vi "Cmd_U32U32U32U32U32U32U32U32U8.vi"(0 "VISA Refnum in":refnum<visa-resource-name>, 1 "Arg1":u32 max=127 step=1, 2 "Arg2":u32 max=127 step=1, 3 "Arg3":u32, 5 "Address":u8, 7 "Cmd":u8, 8 "Arg4":u32, 9 "Arg9":u8, 10 "Arg5":u32, 11 "error in (no error)":errorcluster, 12 "Arg8":u32, 13 "Arg7":u32, 14 "Arg6":u32) -> (4 "VISA Refnum out":refnum<visa-resource-name>, 6 "Valid":bool, 15 "error out":errorcluster)   [LabVIEW 2015, in "Ion Motion Roboclaw.lvlib"]
uses:
  <instrlib>/Ion Motion Roboclaw/Ion Motion Roboclaw.lvlib
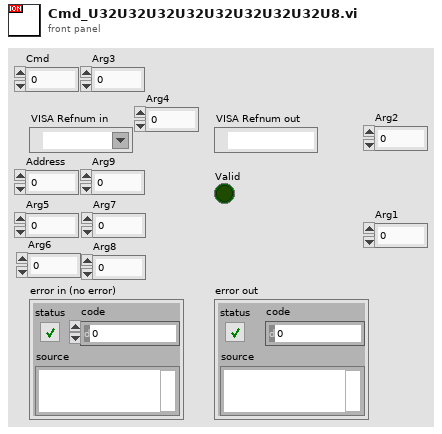
[diagram p1: front panel]
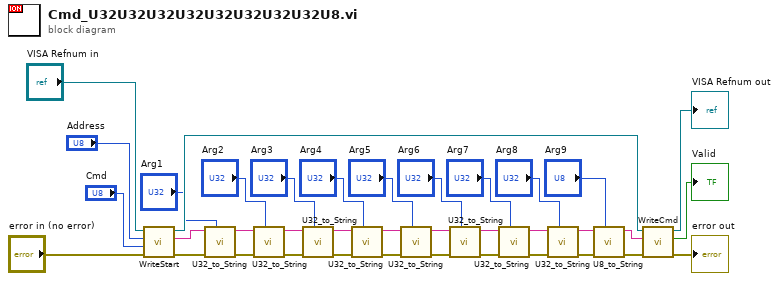
[diagram p0: block diagram]
diagram:
  n1 = call <instrlib>:"WriteStart.vi"("error in (no error)"="error in (no error)", "Cmd"="Cmd", "Address"="Address", "VISA Refnum in"="VISA Refnum in") -> ("error out"=w29:errorcluster, "String Out"=w30:string, "VISA Refnum out"=w32:refnum<visa-resource-name>)  [unwired: 5 in]
  n2 = call <instrlib>:"U32_to_String.vi"("number"="Arg1", "error in (no error)"=w29, "String In"=w30) -> ("error out"=w28:errorcluster, "String Out"=w27:string)  [unwired: 5 in]
  n3 = call <instrlib>:"U32_to_String.vi"("number"="Arg2", "error in (no error)"=w28, "String In"=w27) -> ("error out"=w22:errorcluster, "String Out"=w23:string)  [unwired: 5 in]
  n4 = call <instrlib>:"U32_to_String.vi"("number"="Arg3", "error in (no error)"=w22, "String In"=w23) -> ("error out"=w20:errorcluster, "String Out"=w19:string)  [unwired: 5 in]
  n5 = call <instrlib>:"U32_to_String.vi"("number"="Arg4", "error in (no error)"=w20, "String In"=w19) -> ("error out"=w13:errorcluster, "String Out"=w14:string)  [unwired: 5 in]
  n6 = call <instrlib>:"U32_to_String.vi"("number"="Arg5", "error in (no error)"=w13, "String In"=w14) -> ("error out"=w10:errorcluster, "String Out"=w11:string)  [unwired: 5 in]
  n7 = call <instrlib>:"U32_to_String.vi"("number"="Arg6", "error in (no error)"=w10, "String In"=w11) -> ("error out"=w5:errorcluster, "String Out"=w8:string)  [unwired: 5 in]
  n8 = call <instrlib>:"U32_to_String.vi"("number"="Arg7", "error in (no error)"=w5, "String In"=w8) -> ("error out"=w4:errorcluster, "String Out"=w7:string)  [unwired: 5 in]
  n9 = call <instrlib>:"U32_to_String.vi"("number"="Arg8", "error in (no error)"=w4, "String In"=w7) -> ("error out"=w3:errorcluster, "String Out"=w6:string)  [unwired: 5 in]
  n10 = call <instrlib>:"U8_to_String.vi"("Argument"="Arg9", "error in (no error)"=w3, "String In"=w6) -> ("error out"=w16:errorcluster, "String Out"=w17:string)  [unwired: 5 in]
  n11 = call <instrlib>:"WriteCmd.vi"("error in (no error)"=w16, "write buffer"=w17, "VISA Refnum in"=w32) -> ("error out"=→"error out":errorcluster, "Valid"=→"Valid":bool, "VISA Refnum out"=→"VISA Refnum out":refnum<visa-resource-name>)  [unwired: 2 in]
